vi "Theta(Transmission) (SubVI).vi"(3 "Transmission":dbl, 8 "ParameterA":dbl=0.997938844220231, 10 "ParameterB":dbl=1.035346678618637e-36, 12 "ParameterC":dbl=2.6797703442087277, 14 "ParameterPhi":dbl=38.36882237534376) -> (23 "Position_calcul":dbl=1.0 caption="Position out")   [LabVIEW 2017]
doc: "by Tanguy BOULARD"
panel:
  out "variable en sortie":dbl
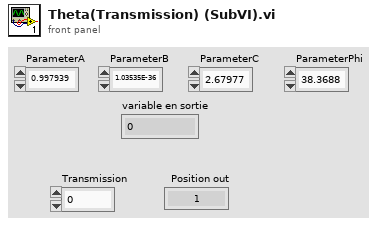
[diagram p1: front panel]
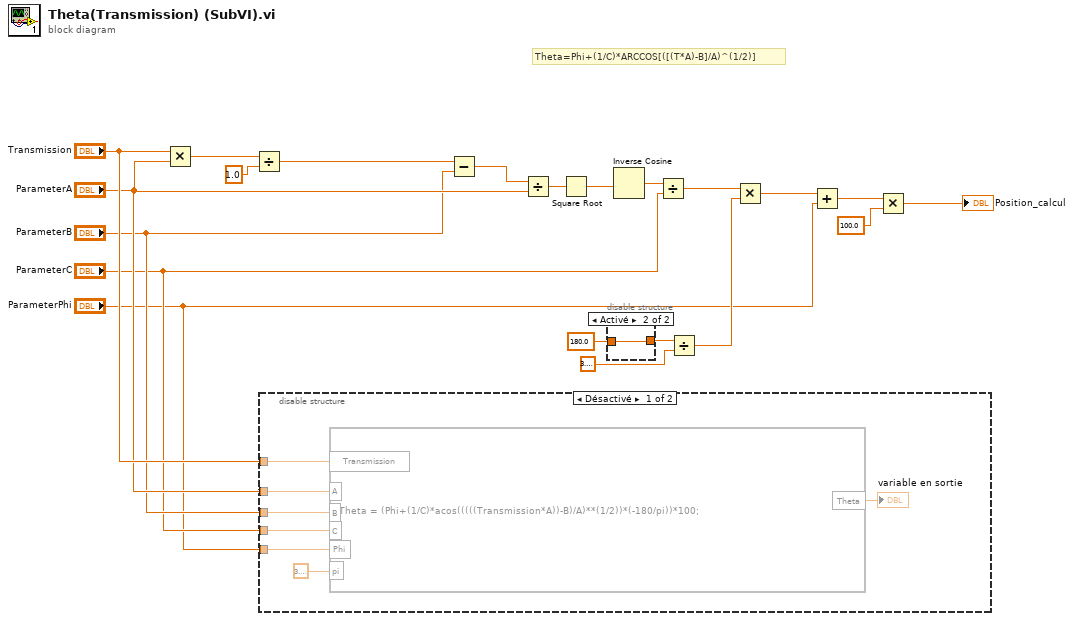
[diagram p0: block diagram]
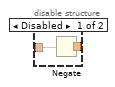
[diagram p3: hidden frame]
diagram:
  # "Theta=Phi+(1/C)*ARCCOS[([(T*A)-B]/A)^(1/2)]"
  n1 = Multiply(x="Transmission", y="ParameterA") -> (x*y=w9:dbl)
  n2 = Divide(x=w9, y=1.0) -> (x/y=w8:dbl)
  n3 = disable-structure shown="Désactivé" {
    disable-tunnel: "Transmission" -> [w28 _]
    disable-tunnel: "ParameterA" -> [w27 _]
    disable-tunnel: "ParameterB" -> [w26 _]
    disable-tunnel: "ParameterC" -> [w25 _]
    disable-tunnel: "ParameterPhi" -> [w24 _]
    frame Disabled {
      n4 = formula code="Theta = (Phi+(1/C)*acos(((((Transmission*A))-B)/A)**(1/2))*(-180/pi))*100;"("Transmission"=w28, "A"=w27, "B"=w26, "C"=w25, "Phi"=w24, "pi"=3.141592653589793) -> ("Theta"=→"variable en sortie":dbl)
    }
    frame Enabled {
    }
  }
  n5 = Subtract(x=w8, y="ParameterB") -> (x-y=w20:dbl)
  n6 = Divide(x=w20, y="ParameterA") -> (x/y=w19:dbl)
  n7 = Square Root(x=w19) -> (sqrt(x)=w17:dbl)
  n8 = disable-structure shown="Activé" {
    disable-tunnel: 180.0 -> [w30 w31]
    disable-tunnel: [w29 w31] -> w6
    frame Disabled {
      n9 = Negate(x=w30) -> (-x=w29:dbl)
    }
    frame Enabled {
    }
  }
  n10 = Inverse Cosine(1:w17) -> (0:w18:dbl)
  n11 = Divide(x=w18, y="ParameterC") -> (x/y=w15:dbl)
  n12 = Divide(x=w6, y=3.141592653589793) -> (x/y=w13:dbl)
  n13 = Multiply(x=w15, y=w13) -> (x*y=w16:dbl)
  n14 = Add(x=w16, y="ParameterPhi") -> (x+y=w12:dbl)
  n15 = Multiply(x=w12, y=100.0) -> (x*y=→"Position_calcul":dbl)
